vi "GetAxisName.vi"(8 "error in (no error)":errorcluster, 10 "axis index":i32, 11 "controller in":refnum<k24>) -> (0 "error out":errorcluster, 2 "axis name":string, 3 "controller out":refnum<k24>)   [LabVIEW 2010]
uses:
  c:/aerotech/controller/stable/A3200/pc/labview/2010/bin/Aerotech.A3200.dll
  bin/Aerotech.A3200.dll
  c:/aerotech/controller/stable/A3200/pc/labview/2010/bin/Aerotech.A3200.LabVIEW.dll
  bin/Aerotech.A3200.LabVIEW.dll
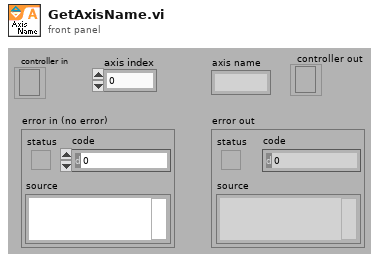
[diagram p1: front panel]
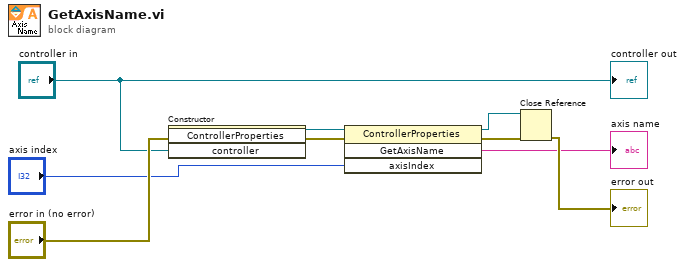
[diagram p0: block diagram]
diagram:
  n1 = constructor class="ControllerProperties"(error in="error in (no error)", "controller"="controller in") -> (reference out=w7:refnum<k24>, error out=w6:errorcluster)  [unwired: 2 in, 2 out]
  n2 = invoke class="ControllerProperties" method="GetAxisName"(reference=w7, error in=w6, "axisIndex"="axis index") -> (reference out=w5:refnum<k24>, error out=w4:errorcluster, "GetAxisName"=→"axis name":string)  [unwired: 1 in, 1 out]
  n3 = Close Reference(reference=w5, error in (no error)=w4) -> (error out=→"error out":errorcluster)
  "controller out" <- "controller in"
